vi "Tosca-Trace-Make Log Entry.vi"(0 "Message":string, 2 "Event":T1, 7 "Value":dbl, 11 "error in (no error)":errorcluster) -> (15 "error out":errorcluster)   [LabVIEW 2020]
uses:
  Tosca-Trace-Event.ctl
  Tosca-Trace Data.ctl
  <vilib>/Utility/error.llb/Error Cluster From Error Code.vi
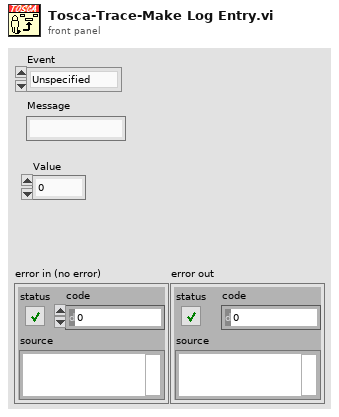
[diagram p1: front panel]
types:
  T1 = typedef "Tosca-Trace-Event.ctl" = enum16{"Unspecified", "Trial start", "Enqueue", "Result", "End parser", "Frame", "Queue available", "Timeout sent", "WritePos", "TTL"}
  T2 = typedef "Tosca-Trace Data.ctl" = cluster{"Time":dbl, "Event":T1, "Source":string, "Message":string, "Data":dbl}
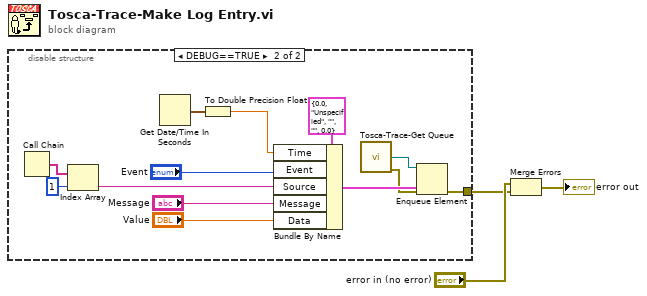
[diagram p0: block diagram]
diagram:
  n1 = disable-structure shown="DEBUG==TRUE" {
    disable-tunnel: [_ w11] -> w1
    frame condition #0 {
    }
    frame condition #1 (active) {
      n2 = Call Chain() -> (call chain=w10:string[])
      n3 = Index Array(array=w10, index=1) -> (element=w9:string)
      n4 = Get Date/Time In Seconds() -> (seconds since 1Jan1904=w6:timestamp)
      n5 = To Double Precision Float(number=w6) -> (double precision float=w5:dbl)
      n6 = Bundle By Name(cluster=T2 {"Time"=0.0, "Event"=enum."Unspecified", "Source"="", "Message"="", "Data"=0.0} ("Trace Data"), "Time"=w5, "Event"="Event", "Source"=w9, "Message"="Message", "Data"="Value") -> (w13:T2)
      n7 = call "Tosca-Trace-Get Queue.vi"() -> ("Trace Queue"=w12:refnum<queue>, "error out"=w4:errorcluster)  [unwired: 14 in]
      n8 = Enqueue Element(queue=w12, element=w13, error in (no error)=w4) -> (error out=w11:errorcluster)  [unwired: 1 in, 2 out]
    }
  }
  n9 = Merge Errors("error in (no error)", w1) -> (→"error out":errorcluster)
